vi "Get occupied squares by color.vi"(8 "error in (no error)":errorcluster, 10 "Color":T4, 11 "Board in":refnum<class "Board.lvclass">) -> (0 "error out":errorcluster, 2 "Squares":T1[](array[typedef]), 3 "Board out":refnum<class "Board.lvclass">)   [LabVIEW 2016, in "Chesslib.lvlib" / "Board.lvclass"]
uses:
  Board.lvclass
  typedef/Color.ctl
  typedef/Square.ctl
  typedef/File.ctl
  typedef/Rank.ctl
  Board.lvclass/Board.ctl
  Pieces/Piece/Piece.lvclass/Piece.ctl
  Pieces/Piece/Piece.lvclass
  Chesslib.lvlib
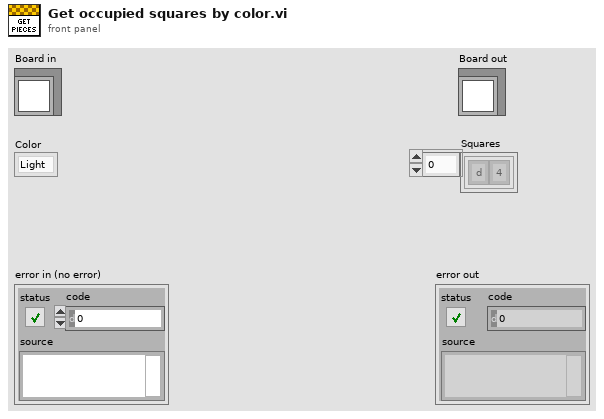
[diagram p1: front panel]
types:
  T1 = typedef "Chesslib.lvlib/Square.ctl" = cluster{"File":T2, "Rank":T3}
  T2 = typedef "Chesslib.lvlib/File.ctl" = enum8{"a", "b", "c", "d", "e", "f", "g", "h"}
  T3 = typedef "Chesslib.lvlib/Rank.ctl" = enum8{"1", "2", "3", "4", "5", "6", "7", "8"}
  T4 = typedef "Chesslib.lvlib/Color.ctl" = enum16{"Light", "Dark"}
  T5 = typedef "Chesslib.lvlib/Board.lvclass/Square content.ctl" = cluster{"Occupied":bool, "Piece":refnum<class "Piece.lvclass">}
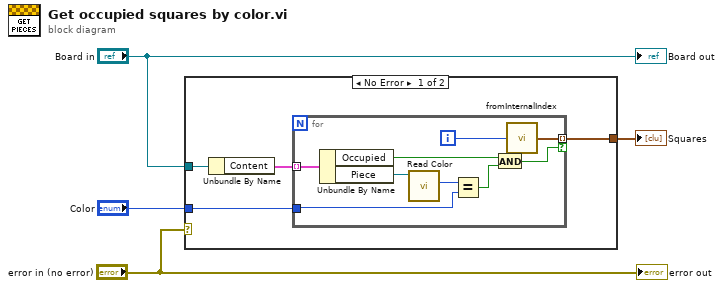
[diagram p0: block diagram]
diagram:
  n1 = case shown="No Error" "error in (no error)" {
    tunnel: "Board in" -> [w8 _]
    tunnel: "Color" -> [w6 _]
    tunnel: [w5 _] -> w2
    frame No Error {
      n2 = Unbundle By Name(w8) -> ("Content"=w7:T5[])
      n3 = for {
        tunnel: w7 -> [w17] mode=indexing
        tunnel: w6 -> [w10]
        tunnel: [w12] -> w5 mode=indexing if=w13
        i -> [w14]
        n4 = Unbundle By Name(w17) -> ("Occupied"=w15:bool, "Piece"=w16:refnum<class "Piece.lvclass">)
        n5 = call "Read Color.vi"("Piece in"=w16) -> ("Color"=w9:T4)  [unwired: 10 in]
        n6 = Equal?(x=w9, y=w10) -> (x = y?=w11:bool)
        n7 = And(x=w15, y=w11) -> (x .and. y?=w13:bool)
        n8 = call "fromInternalIndex.vi"("Internal index"=w14) -> ("Square"=w12:T1)
      }
    }
    frame Error {
    }
  }
  "Squares" <- w2
  "Board out" <- "Board in"
  "error out" <- "error in (no error)"
